vi "HP3458A Config Panel.vi"(8 "error in (no error)":errorcluster, 11 "HP3458A session in":T1={"VISA"="", "ac method"=0, " resolution"=enum."4.5", "function"=0, "frequency source"=0, "auto range"=1, "manual range"=1.0} {"manual range" format="%_3g"; "auto range" items=["OFF", "ON", "ONCE"]; "frequency source" items=["AC + DC Current", "AC + DC Voltage", "AC Current", "AC Voltage"]; "function" items=["DC Voltage", "AC Voltage", "AC + DC Voltage", "DC Current", "AC Current", "AC + DC Current", "2-Wire Resistance", "4-Wire Resistance", "Frequency", "Period", "Direct Sampling DC", "Direct Sampling AC", "Sub-Sampling DC", "Sub-Sampling AC"]; "ac method" items=["Analog", "Random", "Synchronous"]}) -> (0 "error out":errorcluster, 3 "HP3458A session out":T1={"VISA"="", "ac method"=0, " resolution"=enum."4.5", "function"=0, "frequency source"=0, "auto range"=1, "manual range"=1.0} {"manual range" format="%_3g"; "auto range" items=["OFF", "ON", "ONCE"]; "frequency source" items=["AC + DC Current", "AC + DC Voltage", "AC Current", "AC Voltage"]; "function" items=["DC Voltage", "AC Voltage", "AC + DC Voltage", "DC Current", "AC Current", "AC + DC Current", "2-Wire Resistance", "4-Wire Resistance", "Frequency", "Period", "Direct Sampling DC", "Direct Sampling AC", "Sub-Sampling DC", "Sub-Sampling AC"]; "ac method" items=["Analog", "Random", "Synchronous"]})   [LabVIEW 2020]
doc: "Config panel of ACMS Fluke 5790."
uses:
  HP3458A Session.ctl
panel:
  in  "Manual range":dbl=1.0 format="%_3g"
  in  "Auto range":u16(ring)=1 items=["OFF", "ON", "ONCE"]
  in  "Resolution":u16(ring)=2 items=["4.5", "5.5", "6.5", "7.5", "8.5"]
  in  "Frequency source":u16(ring)=3 items=["AC + DC Current", "AC + DC Voltage", "AC Current", "AC Voltage"]
  in  "Function":u16(ring) items=["DC Voltage", "AC Voltage", "AC + DC Voltage", "DC Current", "AC Current", "AC + DC Current", "2-Wire Resistance", "4-Wire Resistance", "Frequency", "Period", "Direct Sampling DC", "Direct Sampling AC", "Sub-Sampling DC", "Sub-Sampling AC"]
  in  "AC method":u16(ring) items=["Analog", "Random", "Synchronous"]
  in  "btn test":bool
  in  "btn ok":bool
  in  "VISA":refnum<visa-resource-name>
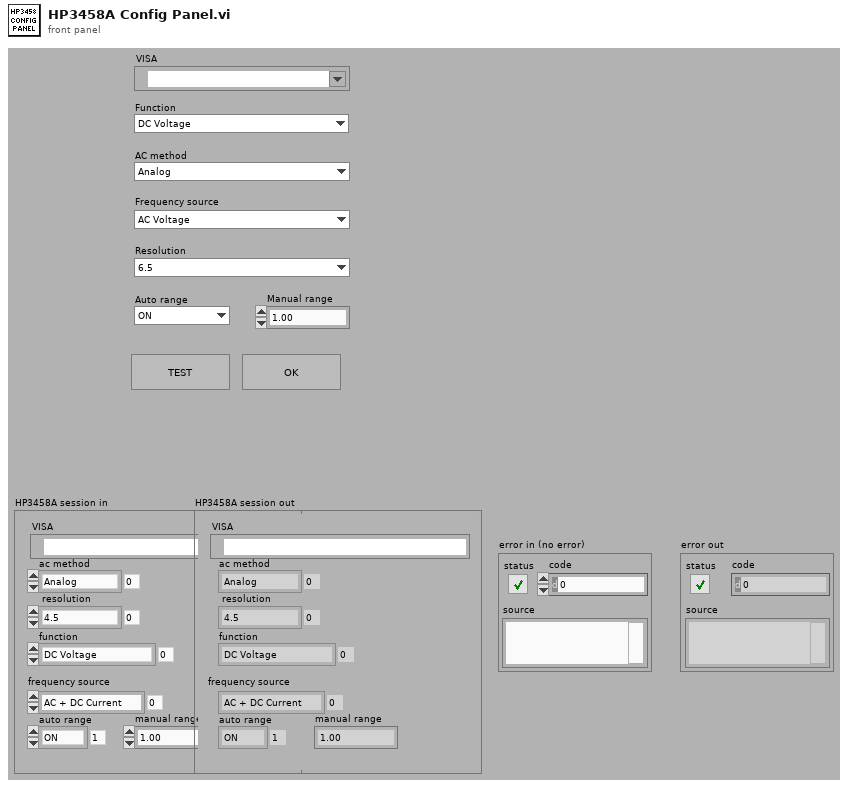
[diagram p1: front panel]
types:
  T1 = typedef "HP3458A Session.ctl" = cluster{"VISA":refnum<visa-resource-name>, "ac method":u16, " resolution":enum16{"4.5", "5.5", "6.5", "7.5", "8.5"}, "function":u16, "frequency source":u16, "auto range":u16, "manual range":dbl}
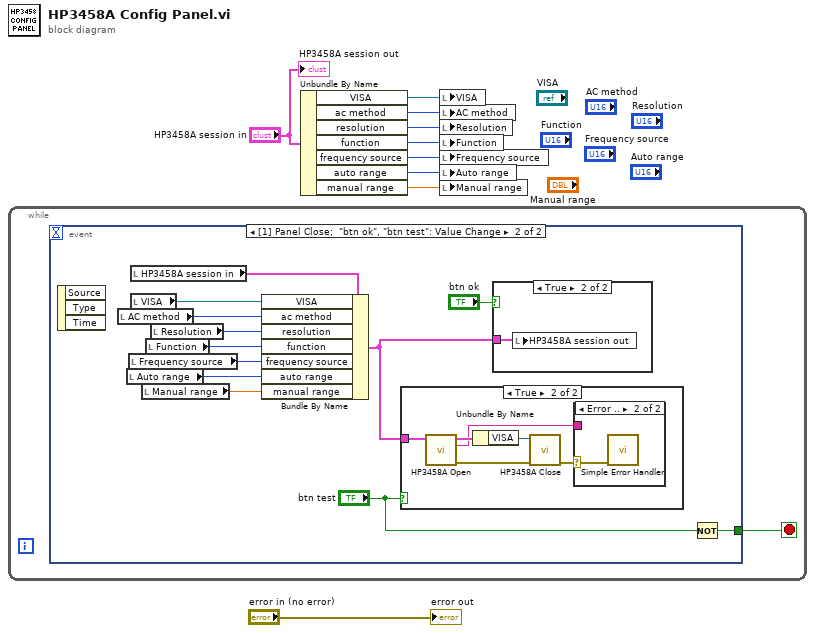
[diagram p0: block diagram]
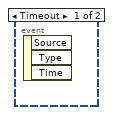
[diagram p2: hidden frame]
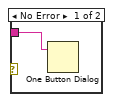
[diagram p4: hidden frame]
diagram:
  n1 = while {
    stop <- w10 stop-if-true
    n2 = event shown="[1] Panel Close;  \"btn ok\", \"btn test\": Value Change" {
      selector: _ -> [_ _]
      dyn-events: _ -> [_ _]
      timeout: _ -> [_ _]
      tunnel: [_ w13] -> w10
      event Timeout {
        n3 = event-data() -> ()  [unwired: 1 in, 3 out]
      }
      event Panel Close; "btn ok", "btn test": Value Change {
        n4 = event-data() -> ()  [unwired: 1 in, 3 out]
        n5 = local read "AC method"() -> (w21:u16)
        n6 = local read "Auto range"() -> (w17:u16)
        n7 = local read "Frequency source"() -> (w18:u16)
        n8 = local read "HP3458A session in"() -> (w16:T1)
        n9 = local read "VISA"() -> (w22:refnum<visa-resource-name>)
        n10 = local read "Manual range"() -> (w11:dbl)
        n11 = local read "Function"() -> (w19:u16)
        n12 = local read "Resolution"() -> (w20:u16)
        n13 = Bundle By Name(cluster=w16, "VISA"=w22, "ac method"=w21, "resolution"=w20, "function"=w19, "frequency source"=w18, "auto range"=w17, "manual range"=w11) -> (w12:T1)
        n14 = case shown="True" "btn test" {
          tunnel: w12 -> [_ w28]
          frame False {
          }
          frame True {
            n15 = call "HP3458A Open.vi"("session in"=w28) -> ("error out"=w27:errorcluster, "idn string"=w23:string, "session out"=w26:T1)  [unwired: 8 in]
            n16 = Unbundle By Name(w26) -> ("VISA"=w25:refnum<visa-resource-name>)
            n17 = call "HP3458A Close.vi"("error in (no error)"=w27, "VISA in"=w25) -> ("error out"=w24:errorcluster)  [unwired: 9 in]
            n18 = case shown="Error .." w24 {
              selector: w24 -> [_ w30]
              tunnel: w23 -> [w29 _]
              frame No Error {
                n19 = One Button Dialog(message=w29) -> ()  [unwired: 1 in, 1 out]
              }
              frame Error {
                n20 = call <vilib>:"Simple Error Handler.vi"("error in (no error)"=w30) -> ()  [unwired: 4 in, 5 out]
              }
            }
          }
        }
        n21 = case shown="True" "btn ok" {
          tunnel: w12 -> [_ w31]
          frame False {
          }
          frame True {
            n22 = local write "HP3458A session out"(w31) -> ()
          }
        }
        n23 = Not(x="btn test") -> (.not. x?=w13:bool)
      }
    }
  }
  n24 = Unbundle By Name("HP3458A session in") -> ("VISA"=w8:refnum<visa-resource-name>, "ac method"=w6:u16, "resolution"=w5:enum16{"4.5", "5.5", "6.5", "7.5", "8.5"}, "function"=w4:u16, "frequency source"=w3:u16, "auto range"=w2:u16, "manual range"=w1:dbl)
  n25 = local write "VISA"(w8) -> ()
  n26 = local write "AC method"(w6) -> ()
  n27 = local write "Resolution"(w5) -> ()
  n28 = local write "Function"(w4) -> ()
  n29 = local write "Frequency source"(w3) -> ()
  n30 = local write "Auto range"(w2) -> ()
  n31 = local write "Manual range"(w1) -> ()
  "HP3458A session out" <- "HP3458A session in"
  "error out" <- "error in (no error)"
